vi "Read Rectifier Recipe.vi"(0 "selected path":path, 11 "error in":errorcluster) -> (1 "Left Amps":dbl[](array[numeric]), 3 "Left AmpMins":dbl[](array[numeric]), 4 "Canceled?":bool, 6 "Num Steps":i32, 8 "name":string, 10 "Rev Mult":dbl, 12 "Right Amps":dbl[](array[numeric]), 14 "Right AmpMins":dbl[](array[numeric]), 15 "error out":errorcluster)   [LabVIEW 2019]
uses:
  <vilib>/Utility/config.llb/Read Key (I32).vi
  <vilib>/Utility/config.llb/Read Key (Double).vi
  <vilib>/Utility/config.llb/NI_LVConfig.lvlib
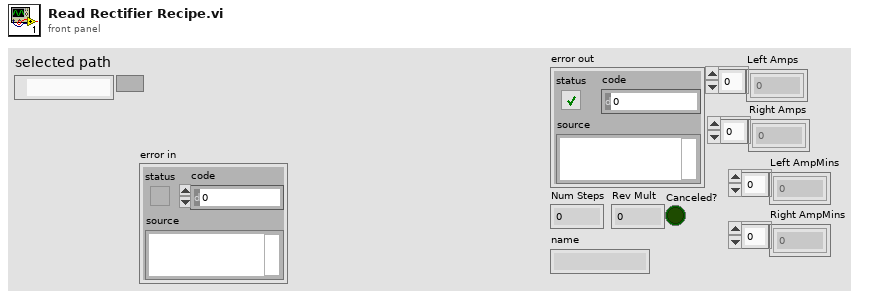
[diagram p1: front panel]
types:
  T1 = typedef "NI_LVConfig.lvlib/Config Data RefNum.ctl" = refnum<k1>
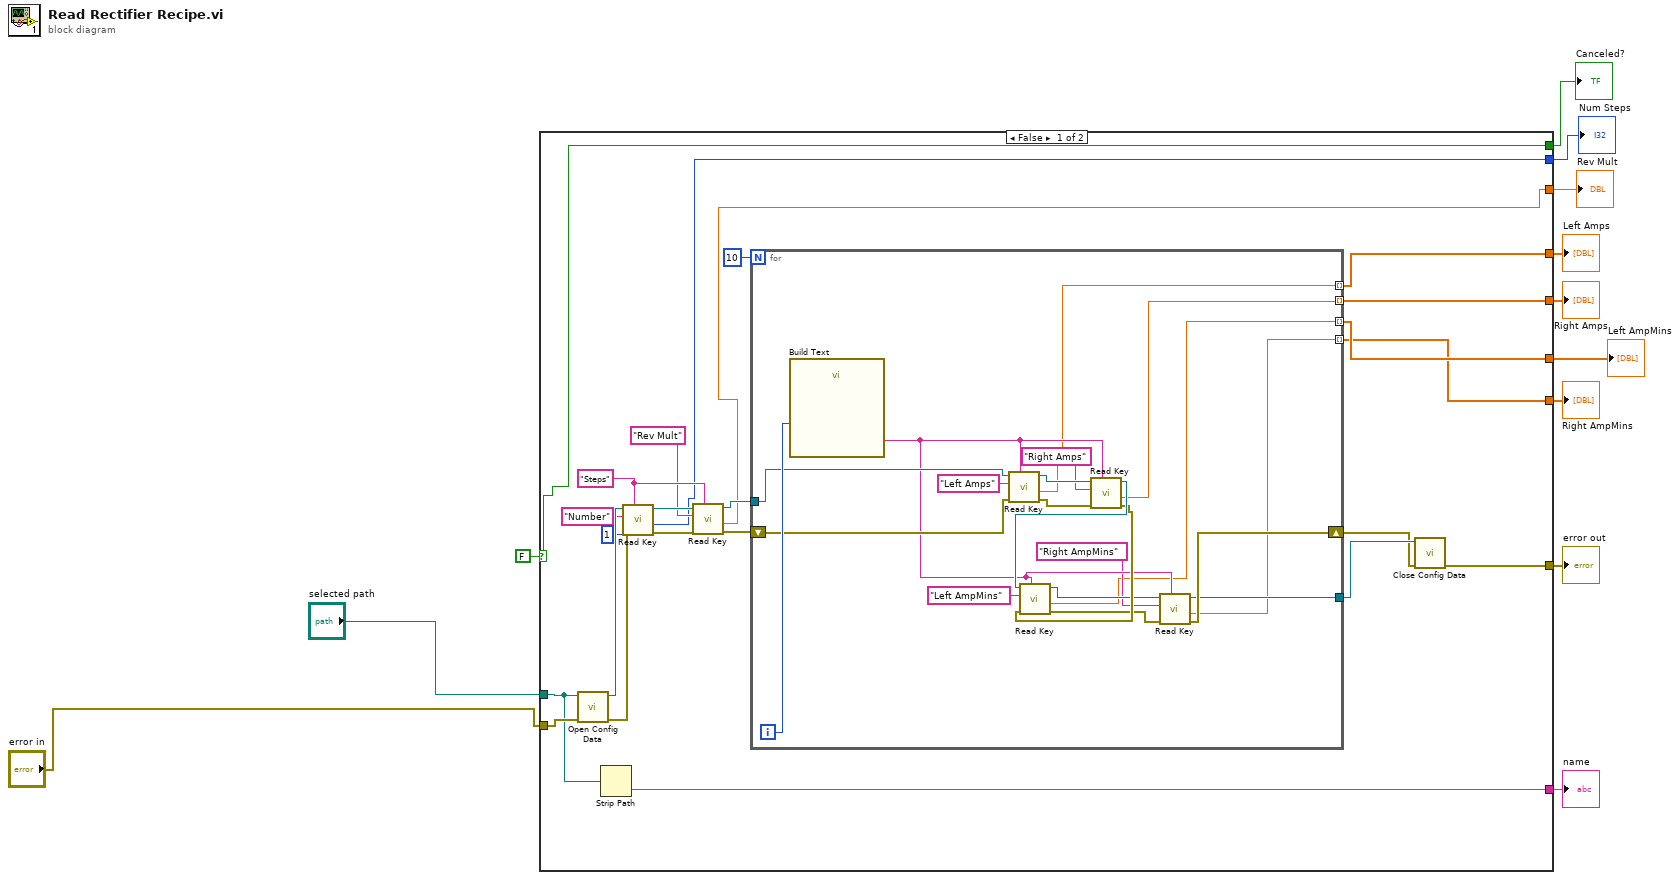
[diagram p0: block diagram]
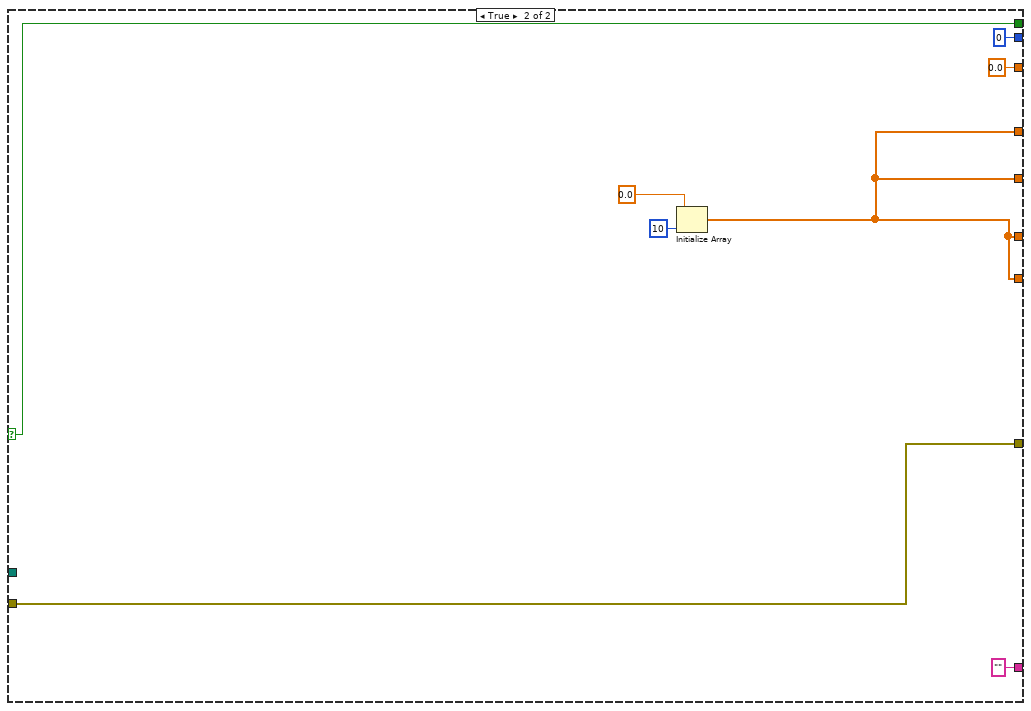
[diagram p2: hidden frame]
diagram:
  n1 = case shown="False" FALSE {
    selector: FALSE -> [w16 w59]
    tunnel: "selected path" -> [w14 _]
    tunnel: "error in" -> [w35 w64]
    tunnel: [w29 w64] -> w12
    tunnel: [w21 0 ("value")] -> w11
    tunnel: [w20 w60] -> w10
    tunnel: [w19 w60] -> w9
    tunnel: [w18 w60] -> w8
    tunnel: [w17 w60] -> w7
    tunnel: [w16 w59] -> w6
    tunnel: [w15 0.0 ("value")] -> w5
    tunnel: [w13 "" ("name")] -> w4
    frame False {
      w26 = "Steps" ("section")
      n2 = call <vilib>:"Open Config Data.vi"("error in (no error)"=w35, "configuration file path"=w14) -> ("error out"=w32:errorcluster, "refnum"=w34:T1)  [unwired: 7 in, 1 out]
      n3 = Strip Path(path=w14) -> (name=w13:string)  [unwired: 1 out]
      n4 = call-poly <vilib>:"Read Key.vi"("section"=w26, "error in (no error)"=w32, "default value"=1, "key"="Number", "refnum"=w34) -> ("error out"=w25:errorcluster, "value"=w21:i32, "refnum out"=w28:T1)  [unwired: 3 in, 1 out]
      n5 = call-poly <vilib>:"Read Key.vi"("section"=w26, "error in (no error)"=w25, "key"="Rev Mult", "refnum"=w28) -> ("error out"=w24:errorcluster, "value"=w15:dbl, "refnum out"=w27:T1)  [unwired: 4 in, 1 out]
      n6 = for {
        N: 10 -> [_]
        tunnel: w27 -> [w54]
        shift-right: [w44] -> w30
        shift-left: w24 -> [w53]
        tunnel: [w41] -> w31
        tunnel: [w40] -> w20 mode=indexing
        tunnel: [w39] -> w19 mode=indexing
        tunnel: [w38] -> w18 mode=indexing
        tunnel: [w37] -> w17 mode=indexing
        i -> [w55]
        n7 = call "Build Text"("d"=w55) -> ("Result"=w43:string)  [unwired: 13 in, 1 out]
        n8 = call-poly <vilib>:"Read Key.vi"("section"=w43, "error in (no error)"=w53, "key"="Left Amps", "refnum"=w54) -> ("error out"=w50:errorcluster, "value"=w40:dbl, "refnum out"=w52:T1)  [unwired: 4 in, 1 out]
        n9 = call-poly <vilib>:"Read Key.vi"("section"=w43, "error in (no error)"=w50, "key"="Right Amps", "refnum"=w52) -> ("error out"=w48:errorcluster, "value"=w39:dbl, "refnum out"=w49:T1)  [unwired: 4 in, 1 out]
        n10 = call-poly <vilib>:"Read Key.vi"("section"=w43, "error in (no error)"=w48, "key"="Left AmpMins", "refnum"=w49) -> ("error out"=w45:errorcluster, "value"=w38:dbl, "refnum out"=w46:T1)  [unwired: 4 in, 1 out]
        n11 = call-poly <vilib>:"Read Key.vi"("section"=w43, "error in (no error)"=w45, "key"="Right AmpMins", "refnum"=w46) -> ("error out"=w44:errorcluster, "value"=w37:dbl, "refnum out"=w41:T1)  [unwired: 4 in, 1 out]
      }
      n12 = call <vilib>:"Close Config Data.vi"("error in (no error)"=w30, "refnum"=w31) -> ("error out"=w29:errorcluster)  [unwired: 8 in, 1 out]
    }
    frame True {
      n13 = Initialize Array(0.0 ("element"), 10 ("dimension size")) -> (w60:dbl[])
    }
  }
  "error out" <- w12
  "Rev Mult" <- w5
  "Num Steps" <- w11
  "Canceled?" <- w6
  "Left Amps" <- w10
  "Right Amps" <- w9
  "Left AmpMins" <- w8
  "Right AmpMins" <- w7
  "name" <- w4
